vi "show selected.vi"(11 "Selected Items (IDs)":string[](array[string])) -> ()   [LabVIEW 2023]
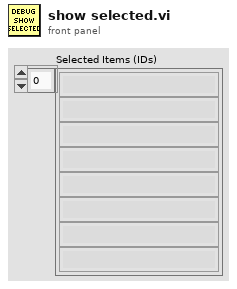
[diagram p1: front panel]
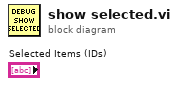
[diagram p0: block diagram]
diagram:
